vi "Config-Meas-Range.vi"(8 "error in (no error)":errorcluster, 9 "zero cancel":bool, 10 "measurement range":T1(array[cluster]) {"unit (VMU1:0)" items=["VMU1", "VMU2", "SMU1", "SMU2", "SMU3", "SMU4", "SMU5", "SMU6"]; "SMU V range\n(2 V:0)" items=["2 V", "20 V", "40 V", "100 V ", "200 V"]; "VMU range\n(2 V:1)" items=["0.2 V", "2 V", "20 V"]; "SMU I range\n(1 nA:2)" items=["10 pA", "100 pA", "1 nA", "10 nA", "100 nA", "1 uA", "10 uA", "100 uA", "1 mA", "10 mA", "100 mA", "1 A"]; "range (fixed:1)" items=["auto", "fixed", "limited"]}, 11 "VISA session":refnum<visa-resource-name>) -> (0 "error out":errorcluster, 3 "VISA resource name out":refnum<visa-resource-name>)   [LabVIEW 2016, in "Agilent 415X Series.lvlib"]
uses:
  Agilent 415X Series.lvlib
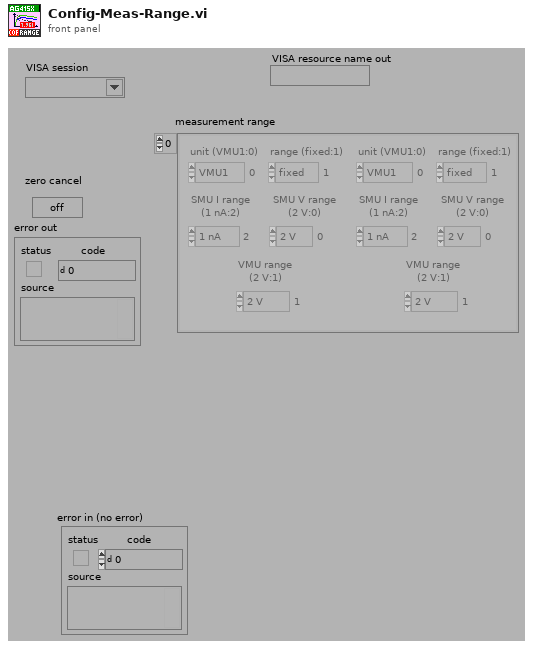
[diagram p1: front panel]
types:
  T1 = cluster{"unit (VMU1:0)":u16, "range (fixed:1)":u16, "SMU I range\n(1 nA:2)":u16, "SMU V range\n(2 V:0)":u16, "VMU range\n(2 V:1)":u16}[]
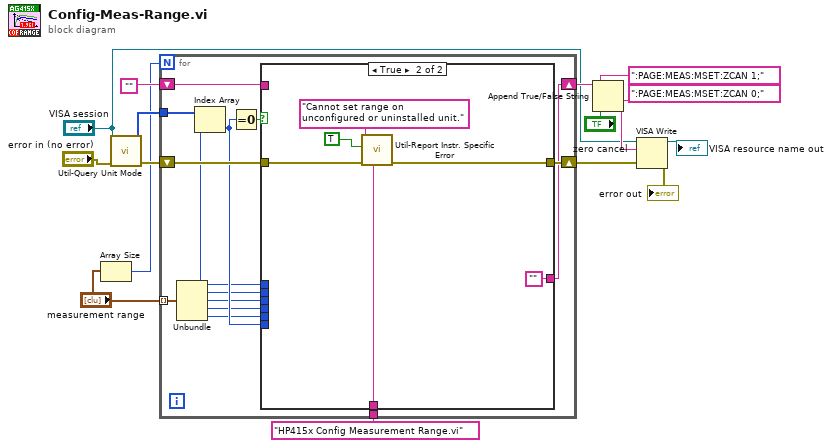
[diagram p0: block diagram]
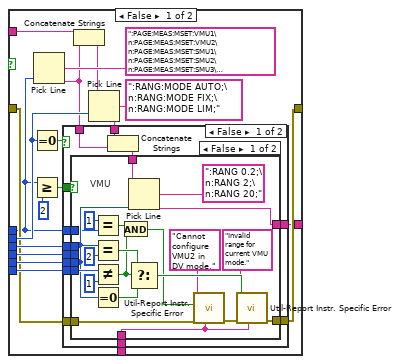
[diagram p2: hidden frame]
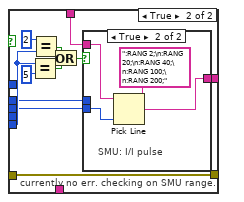
[diagram p3: hidden frame]
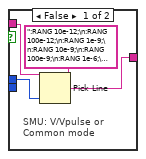
[diagram p4: hidden frame]
diagram:
  n1 = Array Size(array="measurement range") -> (size(s)=w2:i32)
  n2 = call "Util-Query Unit Mode.vi"("error in (no error)"="error in (no error)", "VISA session"="VISA session") -> ("error out"=w14:errorcluster, "unit mode"=w15:u8[])  [unwired: 7 in, 1 out]
  n3 = for {
    N: w2 -> [_]
    tunnel: w15 -> [w29]
    shift-right: [w26] -> w6
    shift-left: w14 -> [w27]
    tunnel: "measurement range" -> [w30] mode=indexing
    tunnel: "HP415x Config Measurement Range.vi" -> [w25]
    shift-right: [w22] -> w10
    shift-left: "" -> [w24]
    n4 = Unbundle(w30) -> ("unit (VMU1:0)"=w21:u16, "range (fixed:1)"=w20:u16, "SMU I range\n(1 nA:2)"=w18:u16, "SMU V range\n(2 V:0)"=w17:u16, "VMU range\n(2 V:1)"=w19:u16)
    n5 = Index Array(array=w29, index=w21) -> (element=w23:u8)
    n6 = Equal To 0?(x=w23) -> (x = 0?=w28:bool)
    n7 = case shown="True" w28 {
      tunnel: w27 -> [w37 w110]
      tunnel: [w36 w109] -> w26
      tunnel: w25 -> [w38 w108]
      tunnel: w20 -> [w46 _]
      tunnel: w18 -> [w44 _]
      tunnel: w17 -> [w43 _]
      tunnel: w19 -> [w42 _]
      tunnel: w21 -> [w31 _]
      tunnel: w24 -> [w34 _]
      tunnel: w23 -> [w41 _]
      tunnel: [w35 ""] -> w22
      frame False {
        n8 = Equal To 0?(x=w46) -> (x = 0?=w45:bool)
        n9 = Greater Or Equal?(x=w31, y=2) -> (x >= y?=w40:bool)
        n10 = Pick Line(multi-line string=":PAGE:MEAS:MSET:VMU1\n:PAGE:MEAS:MSET:VMU2\n:PAGE:MEAS:MSET:SMU1\n:PAGE:MEAS:MSET:SMU2\n:PAGE:MEAS:MSET:SMU3\n:PAGE:MEAS:MSET:SMU4\n:PAGE:MEAS:MSET:SMU5\n:PAGE:MEAS:MSET:SMU6", line index=w31) -> (output string=w33:string)  [unwired: 1 in]
        n11 = Concatenate Strings(w34, w33) -> (w32:string)
        n12 = Pick Line(string ("")=w32, multi-line string=":RANG:MODE AUTO;\n:RANG:MODE FIX;\n:RANG:MODE LIM;", line index=w46) -> (output string=w47:string)
        n13 = case shown="False" w45 {
          tunnel: w47 -> [w59 w104]
          tunnel: w44 -> [w62 _]
          tunnel: w43 -> [w61 _]
          tunnel: w42 -> [w60 _]
          tunnel: w41 -> [w55 _]
          tunnel: w33 -> [w58 _]
          tunnel: w40 -> [w56 _]
          tunnel: w38 -> [w54 _]
          tunnel: w37 -> [w53 w103]
          tunnel: [w52 w103] -> w36
          tunnel: [w51 w104] -> w35
          tunnel: w31 -> [w50 _]
          frame False {
            n14 = Concatenate Strings(w59, w58) -> (w57:string)
            n15 = case shown="False" w56 {
              tunnel: w62 -> [_ w86]
              tunnel: w61 -> [_ w85]
              tunnel: w60 -> [w69 _]
              tunnel: w57 -> [w83 w84]
              tunnel: w55 -> [w81 w87]
              tunnel: w54 -> [w72 _]
              tunnel: w53 -> [w73 w93]
              tunnel: [w77 w93] -> w52
              tunnel: [w75 w94] -> w51
              tunnel: w50 -> [w68 _]
              frame False {
                # "VMU"
                n16 = Equal?(x=1, y=w68) -> (x = y?=w65:bool)
                n17 = Equal?(x=w69, y=2) -> (x = y?=w70:bool)
                n18 = Not Equal?(x=w81, y=1) -> (x != y?=w66:bool)
                n19 = Equal To 0?(x=w69) -> (x = 0?=w71:bool)
                n20 = And(x=w65, y=w66) -> (x .and. y?=w64:bool)
                n21 = Pick Line(string ("")=w83, multi-line string=":RANG 0.2;\n:RANG 2;\n:RANG 20;", line index=w69) -> (output string=w75:string)
                n22 = Select(t=w70, s=w66, f=w71) -> (s? t:f=w78:bool)
                n23 = call "Util-Report Instr. Specific Error.vi"("source"=w72, "error in (no error)"=w73, "error message"="Cannot configure VMU2 in DV mode.", "new error"=w64) -> ("error out"=w74:errorcluster)  [unwired: 6 in, 1 out]
                n24 = call "Util-Report Instr. Specific Error.vi"("source"=w72, "error in (no error)"=w74, "error message"="Invalid range for current VMU mode.", "new error"=w78) -> ("error out"=w77:errorcluster)  [unwired: 6 in, 1 out]
              }
              frame True {
                # "currently no err. checking on SMU range."
                n25 = Equal?(x=w87, y=5) -> (x = y?=w89:bool)
                n26 = Equal?(x=2, y=w87) -> (x = y?=w90:bool)
                n27 = Or(x=w90, y=w89) -> (x .or. y?=w88:bool)
                n28 = case shown="True" w88 {
                  tunnel: [w97 w100] -> w94
                  tunnel: w86 -> [w95 _]
                  tunnel: w85 -> [_ w101]
                  tunnel: w84 -> [w96 w99]
                  frame False {
                    # "SMU: V/Vpulse or\nCommon mode"
                    n29 = Pick Line(string ("")=w96, multi-line string=":RANG 10e-12;\n:RANG 100e-12;\n:RANG 1e-9;\n:RANG 10e-9;\n:RANG 100e-9;\n:RANG 1e-6;\n:RANG 10e-6;\n:RANG 100e-6;\n:RANG 1e-3;\n:RANG 10e-3;\n:RANG 100e-3;\n:RANG 1;", line index=w95) -> (output string=w97:string)
                  }
                  frame True {
                    # "SMU: I/I pulse"
                    n30 = Pick Line(string ("")=w99, multi-line string=":RANG 2;\n:RANG 20;\n:RANG 40;\n:RANG 100;\n:RANG 200;", line index=w101) -> (output string=w100:string)
                  }
                }
              }
            }
          }
          frame True {
            # "auto range"
          }
        }
      }
      frame True {
        n31 = call "Util-Report Instr. Specific Error.vi"("source"=w108, "error in (no error)"=w110, "error message"="Cannot set range on unconfigured or uninstalled unit.", "new error"=TRUE) -> ("error out"=w109:errorcluster)  [unwired: 6 in, 1 out]
      }
    }
  }
  n32 = Append True/False String(1:"zero cancel", 2:":PAGE:MEAS:MSET:ZCAN 0;", 3:":PAGE:MEAS:MSET:ZCAN 1;", 4:w10) -> (0:w5:string)
  n33 = VISA Write(VISA resource name="VISA session", write buffer=w5, error in (no error)=w6) -> (VISA resource name out=→"VISA resource name out":refnum<visa-resource-name>, error out=→"error out":errorcluster)  [unwired: 1 out]
